vi "Add Player.vi"(8 "error in":errorcluster, 10 "Player name":string, 11 "Match in":refnum<class "Match.lvclass">) -> (0 "error out":errorcluster, 3 "Match out":refnum<class "Match.lvclass">)   [LabVIEW 2016, in "Match.lvclass"]
uses:
  Match.lvclass
  Match.lvclass/Match.ctl
  Player/Player.lvclass
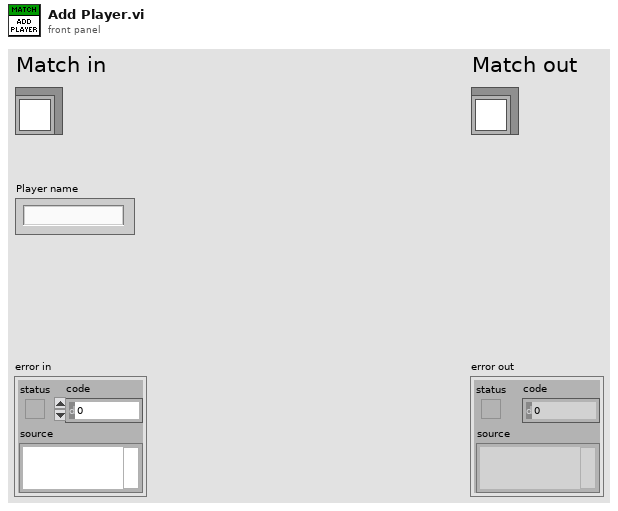
[diagram p1: front panel]
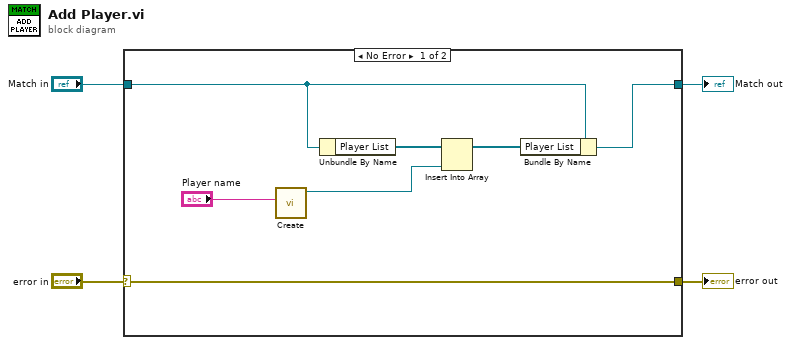
[diagram p0: block diagram]
diagram:
  n1 = case shown="No Error" "error in" {
    selector: "error in" -> [w11 w12]
    tunnel: [w11 w12] -> w3
    tunnel: [w10 w13] -> w1
    tunnel: "Match in" -> [w9 w13]
    frame No Error {
      n2 = call "Create.vi"("Player name"="Player name") -> ("Player.lvclass"=w5:refnum<class "Player.lvclass">)  [unwired: 9 in, 1 out]
      n3 = Unbundle By Name(w9) -> ("Player List"=w8:refnum<class "Player.lvclass">[])
      n4 = Insert Into Array(array=w8, new element=w5) -> (w7:refnum<class "Player.lvclass">[])  [unwired: 1 in]
      n5 = Bundle By Name(cluster=w9, "Player List"=w7) -> (w10:refnum<class "Match.lvclass">)
    }
    frame Error {
    }
  }
  "error out" <- w3
  "Match out" <- w1
